vi "load extension.vi"(7 "pzErrMsg":string, 8 "error in (no error)":errorcluster, 9 "zProc":string, 10 "zFile":string, 11 "db":dbl) -> (0 "error out":errorcluster, 2 "function return":i32, 3 "db out":dbl, 5 "pzErrMsg out":string)   [LabVIEW 2020, in "sqlite3.lvlib"]
uses:
  sqlite3.lvlib
  errstr.vi
  bin/sqlite3_64.dll
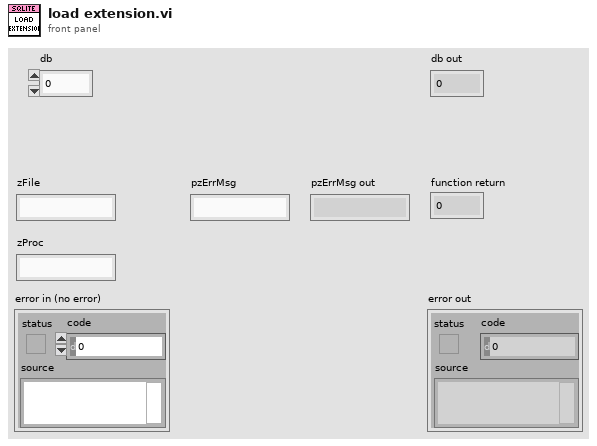
[diagram p1: front panel]
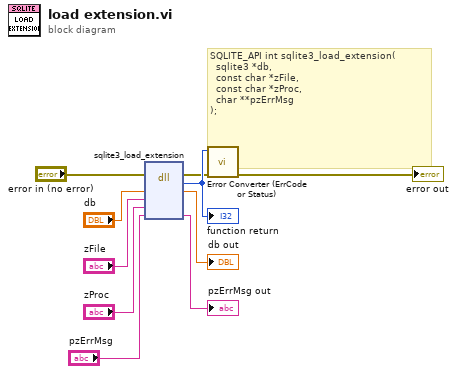
[diagram p0: block diagram]
diagram:
  # "SQLITE_API int sqlite3_load_extension(\n  sqlite3 *db,          \n  const char *zFile,    \n  const char *zProc,    \n  char **pzErrMsg       \n);"
  n1 = dll-call lib="D:/Project/Labview-Projects/database-configuration/externals/sqlite3/Source/bin/sqlite3_*.*" fn="sqlite3_load_extension"(error in="error in (no error)", "db"="db", "zFile"="zFile", "zProc"="zProc", "pzErrMsg"="pzErrMsg") -> (error out=w2:errorcluster, w10:i32, "db"=→"db out":dbl, "pzErrMsg"=→"pzErrMsg out":string)  [unwired: 4 in, 1 out]
  "function return" <- w10
  n2 = call "Error Converter (ErrCode or Status).vi"("error in (no error)"=w2, "error code"=w10) -> ("error out"=→"error out":errorcluster)  [unwired: 9 in]
